vi "Data Logger DHT to LCD_SD Card.vi"   [LabVIEW 2014]
doc: "This example shows how to set and read the current time from a DS1307 Real-Time Clock (RTC). This RTC is used on the Arduino Datalogger Shield, which also comes equipped with an SD card slot. To set the current time, enable the \"Set\" control and populate the date structure with the current date/time, then download the code first. Then turn off \"Set\" and download again to read the time only. The current date/time will be maintained after power cycle if the battery is installed in the shield."
uses:
  <vilib>/Aledyne-TSXperts/Arduino Compatible Compiler for LabVIEW/Code Generator/Arduino APIs/I2C LCD/LiquidCrystal_I2C write String.vi
  <vilib>/Aledyne-TSXperts/Arduino Compatible Compiler for LabVIEW/Arduino Compatible Compiler for LabVIEW.lvlib
  QwaveSys_Interface/QwaveSys_Interface.lvlib
  QwaveSys_ESP8266/QwaveSys_ESP8266.lvlib
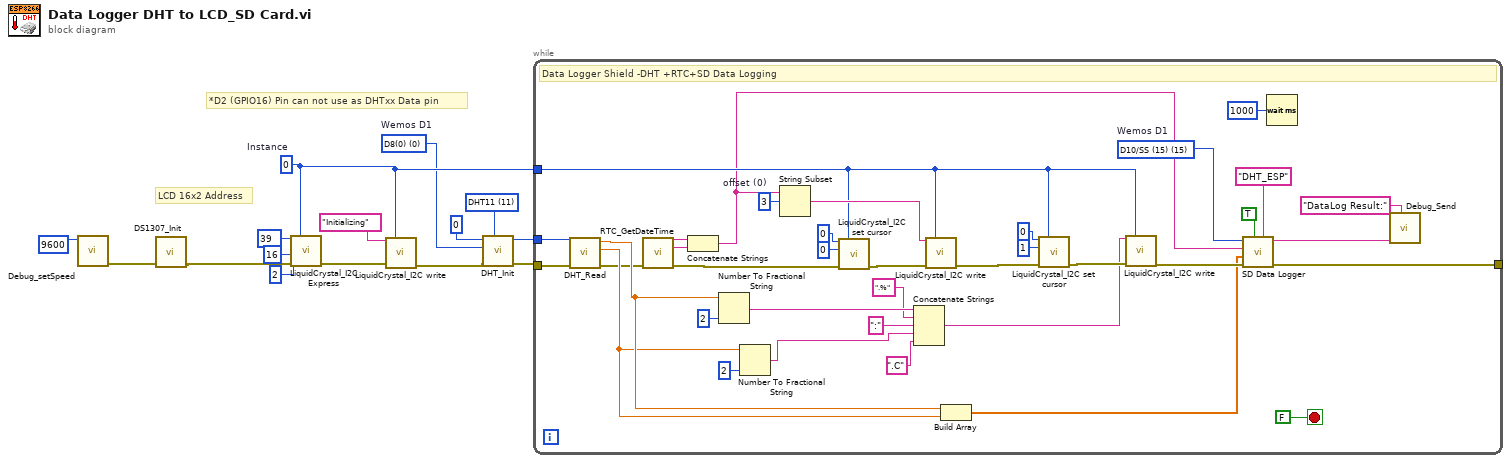
[diagram p0: block diagram]
diagram:
  w5 = u8 0 items=["D0-RX(3)"=3, "D1-TX(1)"=1, "D2(16)"=16, "D3/D15/SCL(5)"=5, "D4/D14/SDA(4)"=4, "D5/D13/SCK(14)-(LED)"=14, "D6/D12/MISO(12)"=12, "D7/D11/MOSI(13)"=13, "D8(0)"=0, "D9/TX1(2)"=2, "D10/SS (15)"=15, "ADC0,(17)"=17]  # Wemos D1
  w7 = u16 11 items=["DHT11"=11, "DHT21"=21, "DHT22"=22] ("Type")
  w10 = u8 0  # Instance
  # "*D2 (GPIO16) Pin can not use as DHTxx Data pin"
  # "LCD 16x2 Address"
  n1 = call "Debug_setSpeed.vi"("Speed"=u32 9600) -> ("error out"=w3:errorcluster)  [unwired: 10 in]
  n2 = call "DS1307_Init.vi"("error in (no error)"=w3) -> ("error out"=w1:errorcluster)  [unwired: 10 in]
  n3 = call <vilib>:"LiquidCrystal_I2C Express.vi"("Addr"=u8 39, "Instance"=w10, "Chars"=u16 16, "Lines"=u16 2, "error in (no error)"=w1) -> ("error out"=w12:errorcluster)  [unwired: 10 in]
  n4 = call-poly <vilib>:"LiquidCrystal_I2C write.vi"("Data"="Initializing", "Instance"=w10, "error in (no error)"=w12) -> ("error out"=w9:errorcluster)  [unwired: 12 in]
  n5 = call "DHT_Init.vi"("Type"=w7, "error in (no error)"=w9, "PIN"=w5, "Interface (0-4)"=u8 0) -> ("error out"=w8:errorcluster, "Instance"=w4:u8)  [unwired: 6 in]
  n6 = while {
    tunnel: w10 -> [w33]
    tunnel: w8 -> [w27]
    tunnel: [w29] -> _
    tunnel: w4 -> [w23]
    stop <- FALSE stop-if-true
    w24 = u8 15 items=["D0-RX(3)"=3, "D1-TX(1)"=1, "D2(16)"=16, "D3/D15/SCL(5)"=5, "D4/D14/SDA(4)"=4, "D5/D13/SCK(14)-(LED)"=14, "D6/D12/MISO(12)"=12, "D7/D11/MOSI(13)"=13, "D8(0)"=0, "D9/TX1(2)"=2, "D10/SS (15)"=15, "ADC0,(17)"=17]  # Wemos D1
    w52 = 3  # offset (0)
    # "Data Logger Shield -DHT +RTC+SD Data Logging"
    n7 = call "DHT_Read.vi"("Instance"=w23, "error in (no error)"=w27) -> ("error out"=w20:errorcluster, "Celsius"=w25:dbl, "Humidity"=w26:dbl)  [unwired: 4 in, 3 out]
    n8 = call "RTC_GetDateTime.vi"("error in (no error)"=w20) -> ("error out"=w19:errorcluster, "time string"=w21:string, "date string"=w22:string)  [unwired: 8 in]
    n9 = Concatenate Strings(w22, w21) -> (w18:string)
    n10 = Number To Fractional String(number=w26, precision (6)=i16 2) -> (F-format string=w39:string)  [unwired: 2 in]
    n11 = Number To Fractional String(number=w25, precision (6)=i16 2) -> (F-format string=w35:string)  [unwired: 2 in]
    n12 = String Subset(string=w18, offset (0)=w52) -> (substring=w49:string)  [unwired: 1 in]
    n13 = call <vilib>:"LiquidCrystal_I2C set cursor.vi"("character"=u16 0, "Instance"=w33, "line"=u16 0, "error in (no error)"=w19) -> ("error out"=w48:errorcluster)  [unwired: 11 in]
    n14 = Concatenate Strings(w39, ".%" ("string"), ":" ("string"), w35, ".C" ("string")) -> (w34:string)
    n15 = call-poly <vilib>:"LiquidCrystal_I2C write.vi"("Data"=w49, "Instance"=w33, "error in (no error)"=w48) -> ("error out"=w42:errorcluster)  [unwired: 12 in]
    n16 = Build Array "Build Array"(w26, w25) -> (w30:dbl[])
    n17 = call <vilib>:"LiquidCrystal_I2C set cursor.vi"("character"=u16 0, "Instance"=w33, "line"=u16 1, "error in (no error)"=w42) -> ("error out"=w45:errorcluster)  [unwired: 11 in]
    n18 = call-poly <vilib>:"LiquidCrystal_I2C write.vi"("Data"=w34, "Instance"=w33, "error in (no error)"=w45) -> ("error out"=w32:errorcluster)  [unwired: 12 in]
    n19 = call <vilib>:"SD Data Logger.vi"("File Name"="DHT_ESP", "Append Timestamp"=TRUE, "error in (no error)"=w32, "Data"=w30, "Timestamp"=w18, "CS Pin"=w24) -> ("error out"=w29:errorcluster, "CSV Data"=w16:string)  [unwired: 4 in]
    n20 = Wait (ms)(milliseconds to wait=u32 1000) -> ()  [unwired: 1 out]
    n21 = call "Debug_Send.vi"("Name"="DataLog Result:", "DATA"=w16) -> ()  [unwired: 10 in]
  }
